vi "Measure Power Sample.vi"() -> ()   [LabVIEW 2019]
panel:
  out "Active":bool
  out "Power Value":dbl caption="Optical Power [W]" format="%#_4p"
  in  "stop":bool
  # "Thorlabs Power Meter Series\n   Measure power example"
  # "This example will connect the first found power meter."
  # "Connected"
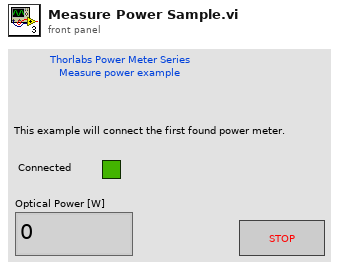
[diagram p1: front panel]
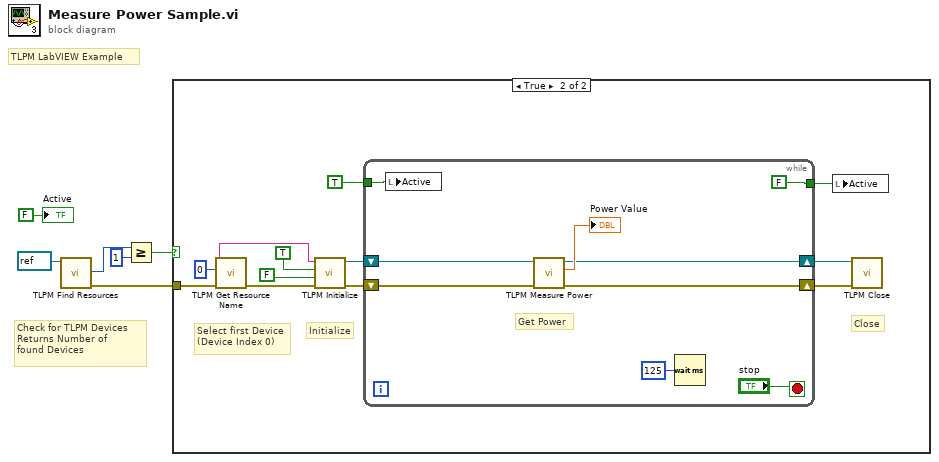
[diagram p0: block diagram]
diagram:
  # "TLPM LabVIEW Example"
  # "Check for TLPM Devices\nReturns Number of\nfound Devices"
  n1 = call <instrlib>:"TLPM Find Resources.vi"("instrument handle"=refnum<visa-resource-name> refnum) -> ("error out"=w5:errorcluster, "Resource Count"=w3:u32)  [unwired: 8 in, 1 out]
  n2 = Greater Or Equal?(x=w3, y=u32 1) -> (x >= y?=w4:bool)
  n3 = case shown="True" w4 {
    tunnel: w5 -> [_ w14]
    frame False {
    }
    frame True {
      # "Close"
      # "Initialize"
      # "Select first Device\n(Device Index 0)"
      n4 = call <instrlib>:"TLPM Get Resource Name.vi"("error in (no error)"=w14, "Index (0)"=u32 0 ("Device Index")) -> ("error out"=w17:errorcluster, "Resource Name"=w15:string)  [unwired: 7 in, 1 out]
      n5 = call <instrlib>:"TLPM Initialize.vi"("error in (no error)"=w17, "Reset Device (Reset Device)"=FALSE ("ID Query (Do Query)"), "ID Query (Do Query)"=TRUE, "resource name"=w15) -> ("error out"=w11:errorcluster, "instrument handle out"=w12:refnum<visa-resource-name>)  [unwired: 6 in]
      n6 = while {
        shift-right: [w20] -> w18
        shift-left: w12 -> [w26]
        shift-right: [w19] -> w16
        shift-left: w11 -> [w25]
        tunnel: [FALSE ("Active")] -> w10
        tunnel: TRUE ("Active") -> [w21]
        stop <- "stop" stop-if-true
        # "Get Power"
        n7 = local write "Active"(w21) -> ()
        n8 = call <instrlib>:"TLPM Measure Power.vi"("error in (no error)"=w25, "instrument handle"=w26) -> ("error out"=w19:errorcluster, "Power"=→"Power Value":dbl, "instrument handle out"=w20:refnum<visa-resource-name>)  [unwired: 7 in]
        n9 = Wait (ms)(milliseconds to wait=u32 125) -> ()  [unwired: 1 out]
      }
      n10 = local write "Active"(w10) -> ()
      n11 = call <instrlib>:"TLPM Close.vi"("error in (no error)"=w16, "instrument handle"=w18) -> ()  [unwired: 9 in, 1 out]
    }
  }
  "Active" <- FALSE ("Active")
